vi "Config_AI_Module_NI.vi"(8 "error in (no error)":errorcluster, 10 "MODULE NAME":string, 11 "Refnum in":refnum<k21>) -> (0 "error out":errorcluster, 3 "Refnum out":refnum<k21>)   [LabVIEW 2019]
uses:
  <vilib>/DAQmx/create/channels.llb/DAQmx Create Channel (AI-Current-Basic).vi
panel:
  out "error out 2":errorcluster
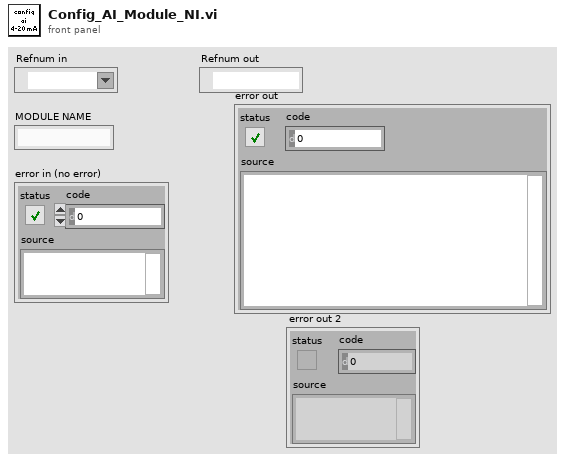
[diagram p1: front panel]
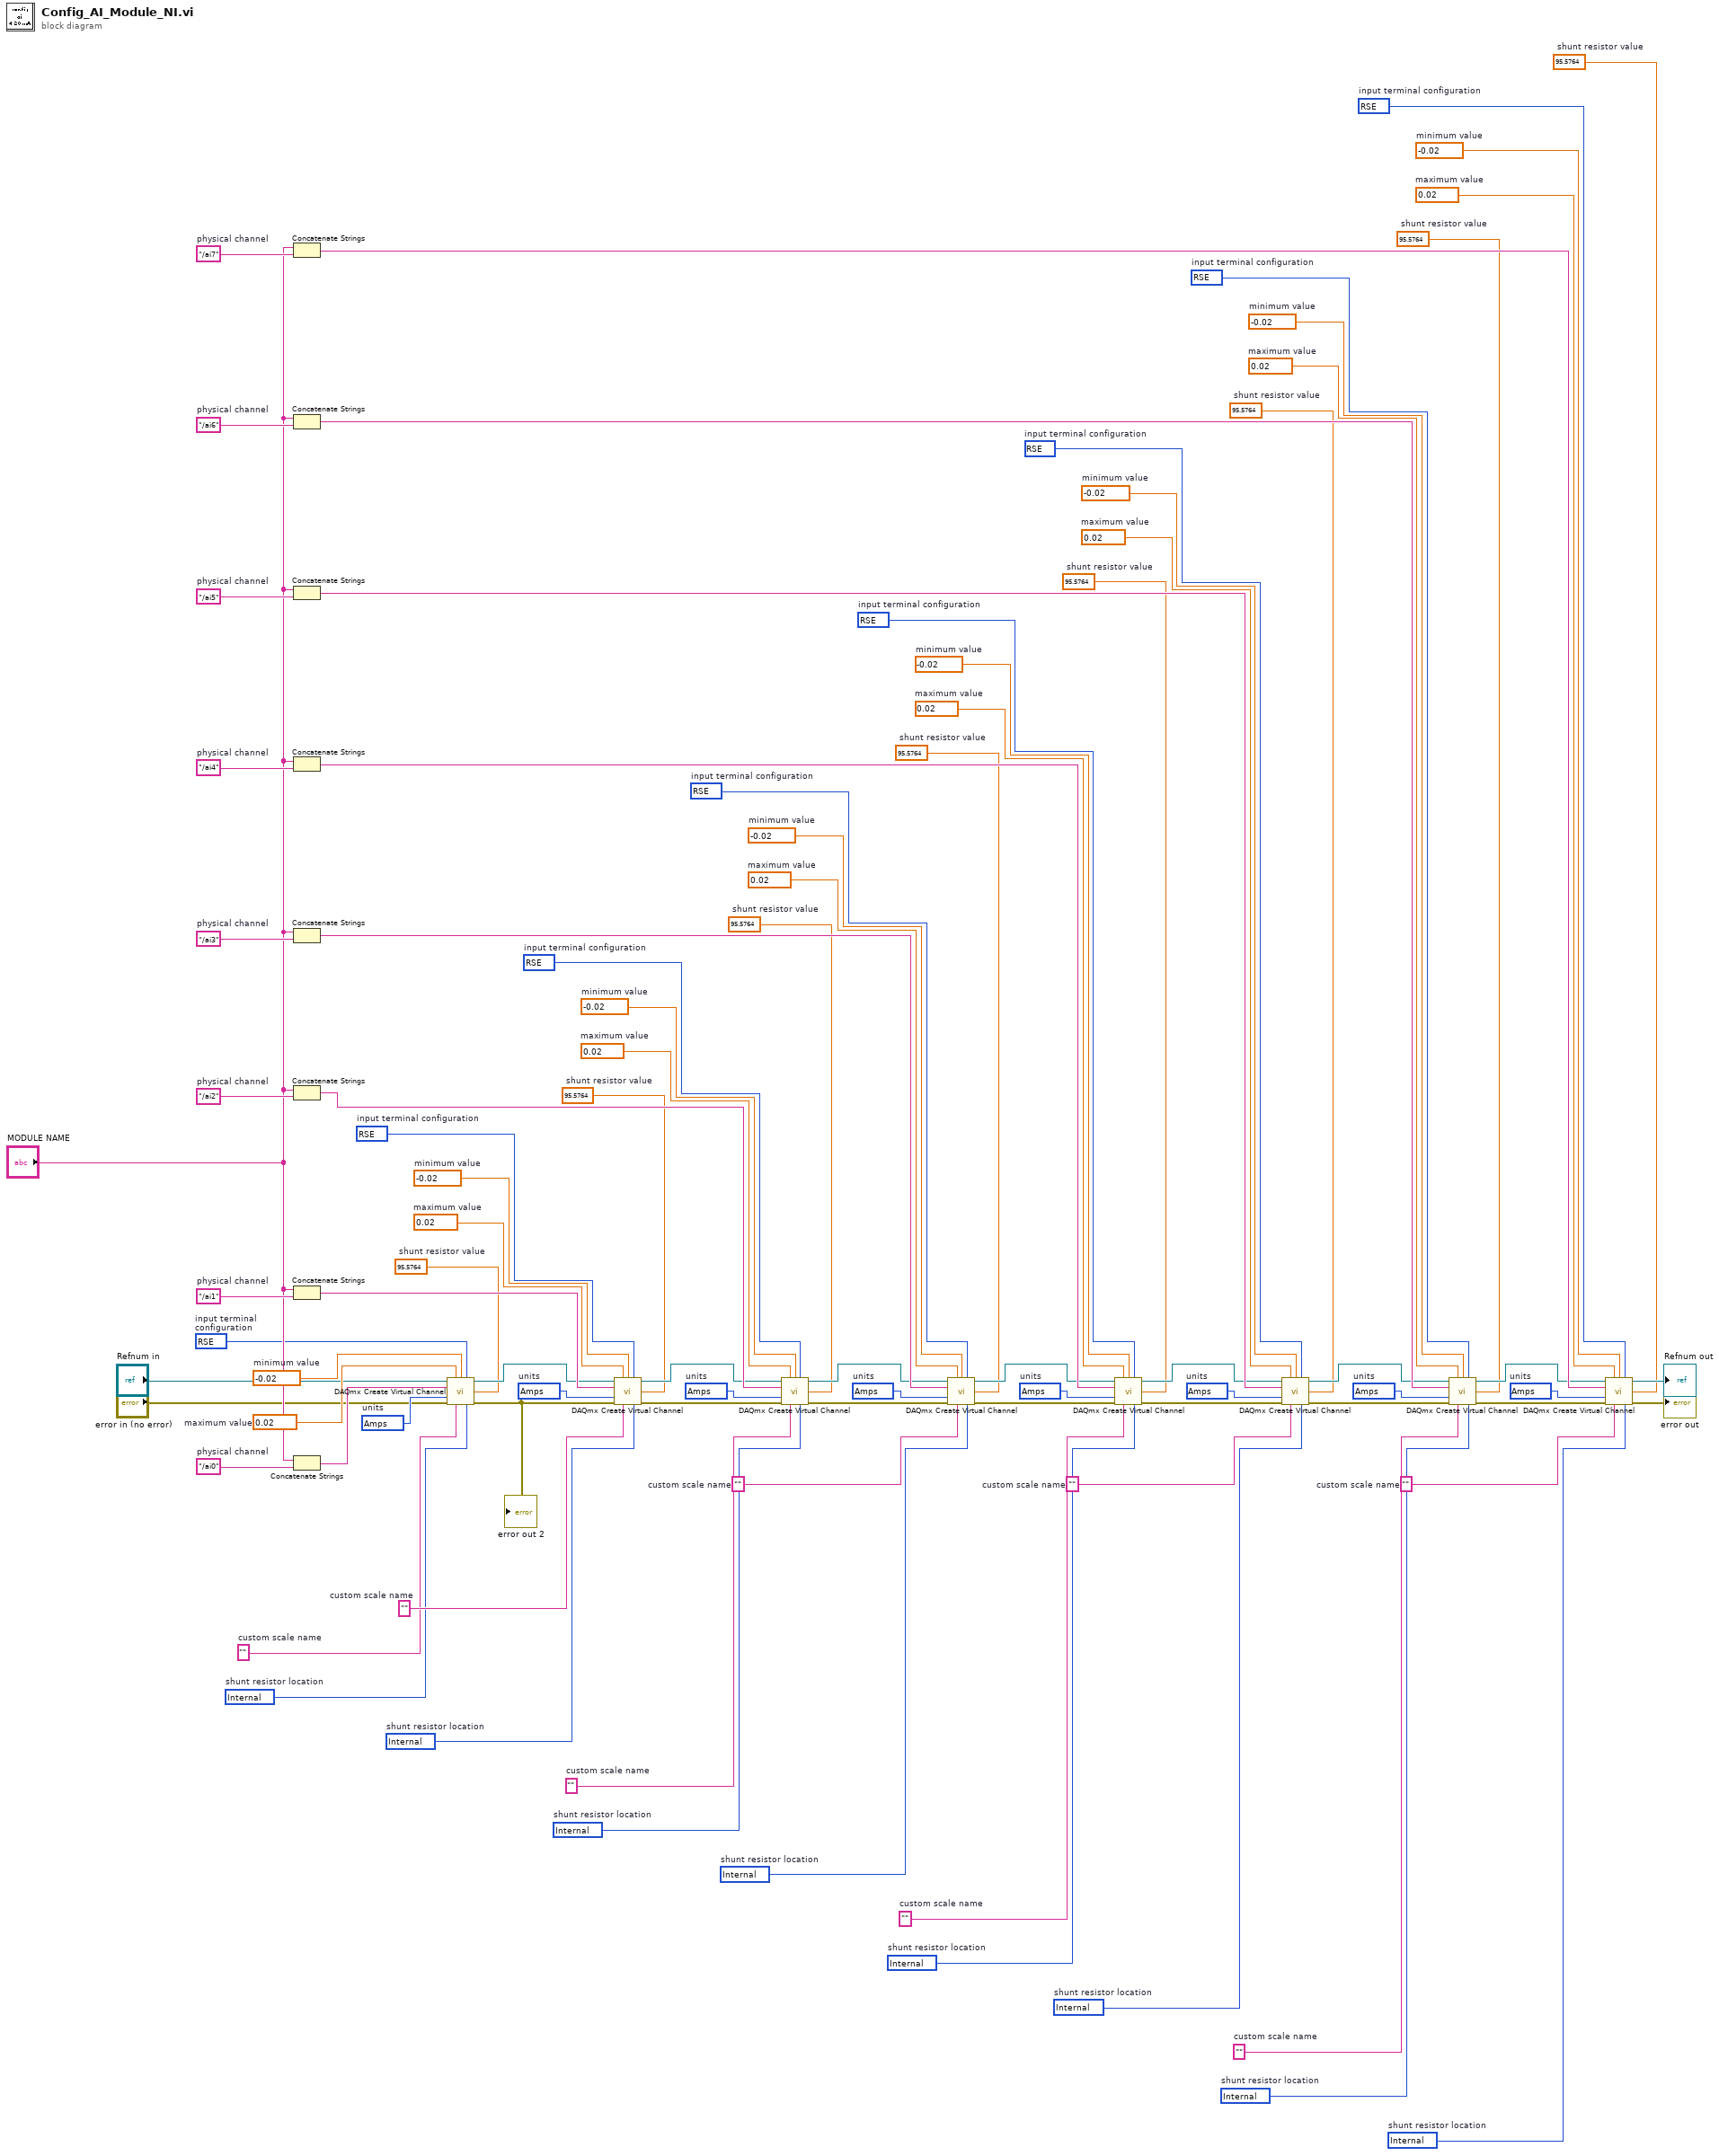
[diagram p0: block diagram]
diagram:
  w72 = 10083 items=["default"=-1, "RSE"=10083, "NRSE"=10078, "Differential"=10106, "Pseudodifferential"=12529]  # input terminal configuration
  w71 = 10342 items=["Amps"=10342, "From Custom Scale"=10065]  # units
  w70 = 95.5764  # shunt resistor value
  w69 = 10200 items=["Internal"=10200, "External"=10167]  # shunt resistor location
  w68 = ""  # custom scale name
  w67 = -0.02  # minimum value
  w66 = 0.02  # maximum value
  w88 = "/ai7"  # physical channel
  w64 = 10083 items=["default"=-1, "RSE"=10083, "NRSE"=10078, "Differential"=10106, "Pseudodifferential"=12529]  # input terminal configuration
  w63 = 10342 items=["Amps"=10342, "From Custom Scale"=10065]  # units
  w62 = 95.5764  # shunt resistor value
  w61 = 10200 items=["Internal"=10200, "External"=10167]  # shunt resistor location
  w59 = ""  # custom scale name
  w58 = -0.02  # minimum value
  w57 = 0.02  # maximum value
  w86 = "/ai6"  # physical channel
  w55 = 10083 items=["default"=-1, "RSE"=10083, "NRSE"=10078, "Differential"=10106, "Pseudodifferential"=12529]  # input terminal configuration
  w54 = 10342 items=["Amps"=10342, "From Custom Scale"=10065]  # units
  w53 = 95.5764  # shunt resistor value
  w52 = 10200 items=["Internal"=10200, "External"=10167]  # shunt resistor location
  w50 = ""  # custom scale name
  w49 = -0.02  # minimum value
  w48 = 0.02  # maximum value
  w84 = "/ai5"  # physical channel
  w46 = 10083 items=["default"=-1, "RSE"=10083, "NRSE"=10078, "Differential"=10106, "Pseudodifferential"=12529]  # input terminal configuration
  w45 = 10342 items=["Amps"=10342, "From Custom Scale"=10065]  # units
  w44 = 95.5764  # shunt resistor value
  w43 = 10200 items=["Internal"=10200, "External"=10167]  # shunt resistor location
  w41 = ""  # custom scale name
  w40 = -0.02  # minimum value
  w39 = 0.02  # maximum value
  w82 = "/ai4"  # physical channel
  w37 = 10083 items=["default"=-1, "RSE"=10083, "NRSE"=10078, "Differential"=10106, "Pseudodifferential"=12529]  # input terminal configuration
  w36 = 10342 items=["Amps"=10342, "From Custom Scale"=10065]  # units
  w35 = 95.5764  # shunt resistor value
  w34 = 10200 items=["Internal"=10200, "External"=10167]  # shunt resistor location
  w32 = ""  # custom scale name
  w31 = -0.02  # minimum value
  w30 = 0.02  # maximum value
  w80 = "/ai3"  # physical channel
  w28 = 10083 items=["default"=-1, "RSE"=10083, "NRSE"=10078, "Differential"=10106, "Pseudodifferential"=12529]  # input terminal configuration
  w27 = 10342 items=["Amps"=10342, "From Custom Scale"=10065]  # units
  w26 = 95.5764  # shunt resistor value
  w25 = 10200 items=["Internal"=10200, "External"=10167]  # shunt resistor location
  w23 = ""  # custom scale name
  w22 = -0.02  # minimum value
  w21 = 0.02  # maximum value
  w78 = "/ai2"  # physical channel
  w19 = 10083 items=["default"=-1, "RSE"=10083, "NRSE"=10078, "Differential"=10106, "Pseudodifferential"=12529]  # input terminal configuration
  w18 = 10342 items=["Amps"=10342, "From Custom Scale"=10065]  # units
  w17 = 95.5764  # shunt resistor value
  w16 = 10200 items=["Internal"=10200, "External"=10167]  # shunt resistor location
  w14 = ""  # custom scale name
  w13 = -0.02  # minimum value
  w12 = 0.02  # maximum value
  w76 = "/ai1"  # physical channel
  w10 = 10083 items=["default"=-1, "RSE"=10083, "NRSE"=10078, "Differential"=10106, "Pseudodifferential"=12529]  # input terminal configuration
  w9 = 10342 items=["Amps"=10342, "From Custom Scale"=10065]  # units
  w8 = 95.5764  # shunt resistor value
  w7 = 10200 items=["Internal"=10200, "External"=10167]  # shunt resistor location
  w5 = ""  # custom scale name
  w4 = -0.02  # minimum value
  w3 = 0.02  # maximum value
  w73 = "/ai0"  # physical channel
  n1 = Concatenate Strings("MODULE NAME", w88) -> (w89:string)
  n2 = Concatenate Strings("MODULE NAME", w86) -> (w87:string)
  n3 = Concatenate Strings("MODULE NAME", w84) -> (w85:string)
  n4 = Concatenate Strings("MODULE NAME", w82) -> (w83:string)
  n5 = Concatenate Strings("MODULE NAME", w80) -> (w81:string)
  n6 = Concatenate Strings("MODULE NAME", w78) -> (w79:string)
  n7 = Concatenate Strings("MODULE NAME", w76) -> (w77:string)
  n8 = Concatenate Strings("MODULE NAME", w73) -> (w74:string)
  n9 = call-poly <vilib>:"DAQmx Create Virtual Channel.vi"("task in"="Refnum in", "maximum value"=w3, "minimum value"=w4, "input terminal configuration"=w10, "physical channels"=w74, "external shunt resistor value"=w8, "units"=w9, "error in"="error in (no error)", "custom scale name"=w5, "shunt resistor location"=w7) -> ("task out"=w11:refnum<k21>, "error out"=w6:errorcluster)  [unwired: 4 in]
  "error out 2" <- w6
  n10 = call-poly <vilib>:"DAQmx Create Virtual Channel.vi"("task in"=w11, "maximum value"=w12, "minimum value"=w13, "input terminal configuration"=w19, "physical channels"=w77, "external shunt resistor value"=w17, "units"=w18, "error in"=w6, "custom scale name"=w14, "shunt resistor location"=w16) -> ("task out"=w20:refnum<k21>, "error out"=w15:errorcluster)  [unwired: 4 in]
  n11 = call-poly <vilib>:"DAQmx Create Virtual Channel.vi"("task in"=w20, "maximum value"=w21, "minimum value"=w22, "input terminal configuration"=w28, "physical channels"=w79, "external shunt resistor value"=w26, "units"=w27, "error in"=w15, "custom scale name"=w23, "shunt resistor location"=w25) -> ("task out"=w29:refnum<k21>, "error out"=w24:errorcluster)  [unwired: 4 in]
  n12 = call-poly <vilib>:"DAQmx Create Virtual Channel.vi"("task in"=w29, "maximum value"=w30, "minimum value"=w31, "input terminal configuration"=w37, "physical channels"=w81, "external shunt resistor value"=w35, "units"=w36, "error in"=w24, "custom scale name"=w32, "shunt resistor location"=w34) -> ("task out"=w38:refnum<k21>, "error out"=w33:errorcluster)  [unwired: 4 in]
  n13 = call-poly <vilib>:"DAQmx Create Virtual Channel.vi"("task in"=w38, "maximum value"=w39, "minimum value"=w40, "input terminal configuration"=w46, "physical channels"=w83, "external shunt resistor value"=w44, "units"=w45, "error in"=w33, "custom scale name"=w41, "shunt resistor location"=w43) -> ("task out"=w47:refnum<k21>, "error out"=w42:errorcluster)  [unwired: 4 in]
  n14 = call-poly <vilib>:"DAQmx Create Virtual Channel.vi"("task in"=w47, "maximum value"=w48, "minimum value"=w49, "input terminal configuration"=w55, "physical channels"=w85, "external shunt resistor value"=w53, "units"=w54, "error in"=w42, "custom scale name"=w50, "shunt resistor location"=w52) -> ("task out"=w56:refnum<k21>, "error out"=w51:errorcluster)  [unwired: 4 in]
  n15 = call-poly <vilib>:"DAQmx Create Virtual Channel.vi"("task in"=w56, "maximum value"=w57, "minimum value"=w58, "input terminal configuration"=w64, "physical channels"=w87, "external shunt resistor value"=w62, "units"=w63, "error in"=w51, "custom scale name"=w59, "shunt resistor location"=w61) -> ("task out"=w65:refnum<k21>, "error out"=w60:errorcluster)  [unwired: 4 in]
  n16 = call-poly <vilib>:"DAQmx Create Virtual Channel.vi"("task in"=w65, "maximum value"=w66, "minimum value"=w67, "input terminal configuration"=w72, "physical channels"=w89, "external shunt resistor value"=w70, "units"=w71, "error in"=w60, "custom scale name"=w68, "shunt resistor location"=w69) -> ("task out"=→"Refnum out":refnum<k21>, "error out"=→"error out":errorcluster)  [unwired: 4 in]
